vi "Get Sub Build Spec.vi"(0 "NI Build Specification in":refnum<class "NI Build Specification_LV.lvclass">, 5 "Sub Build Spec Name":string, 11 "error in (no error)":errorcluster) -> (4 "NI Build Specification out":refnum<class "NI Build Specification_LV.lvclass">, 6 "Sub Build Spec":refnum<class "NI Build Specification_LV.lvclass">, 8 "found":bool, 15 "error out":errorcluster)   [LabVIEW 2017, in "CL_G3_VIComponentBuilder.lvlib" / "NI Build Specification_LV.lvclass"]
doc: "Gets a sub build spec by the name of the build spec in the LabVIEW project."
uses:
  NI Build Specification_LV.lvclass
  NI Build Specification_LV.lvclass/NI Build Specification_LV.ctl
  Accessors/Read Sub Build Specs.vi
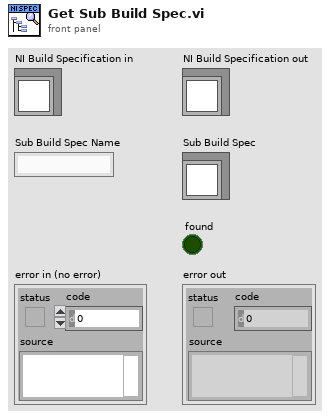
[diagram p1: front panel]
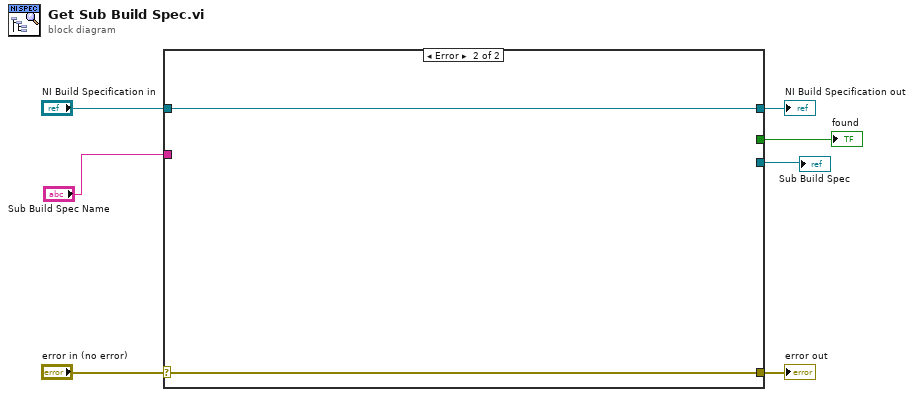
[diagram p0: block diagram]
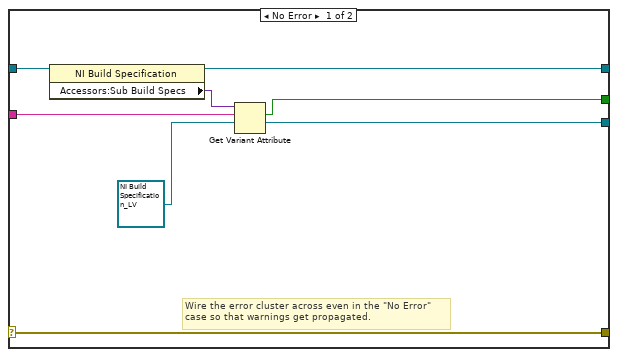
[diagram p2: hidden frame]
diagram:
  n1 = case shown="Error" "error in (no error)" {
    selector: "error in (no error)" -> [w14 w17]
    tunnel: [w14 w17] -> w6
    tunnel: [w13 w16] -> w4
    tunnel: "NI Build Specification in" -> [w15 w16]
    tunnel: "Sub Build Spec Name" -> [w11 _]
    tunnel: [w9 _] -> w2
    tunnel: [w8 _] -> w1
    frame No Error {
      # "Wire the error cluster across even in the \"No Error\"\ncase so that warnings get propagated."
      n2 = property class="NI Build Specification"(reference=w15) -> (reference out=w13:refnum<class "NI Build Specification_LV.lvclass">, "Accessors:Sub Build Specs"=w12:variant)  [unwired: 1 in, 1 out]
      n3 = Get Variant Attribute(Variant=w12, name=w11, default value (empty Variant)=refnum<class "NI Build Specification_LV.lvclass"> refnum ("NI Build Specification in 2")) -> (found=w8:bool, value=w9:refnum<class "NI Build Specification_LV.lvclass">)  [unwired: 1 in, 2 out]
    }
    frame Error {
    }
  }
  "error out" <- w6
  "NI Build Specification out" <- w4
  "Sub Build Spec" <- w2
  "found" <- w1
